vi "Integrl2.vi"(1 "Sampling frequency":i32=1000, 2 "Input Array":dbl[](array[numeric]) format="%.2f") -> (0 "Output Array (Integral)":dbl[](array[numeric]) format="%.2f")   [LabVIEW 2011]
uses:
  <vilib>/Analysis/NI_AALPro.lvlib
panel:
  out "Error":i32
  in  "Final condition":i32
  in  "Initial condition":i32
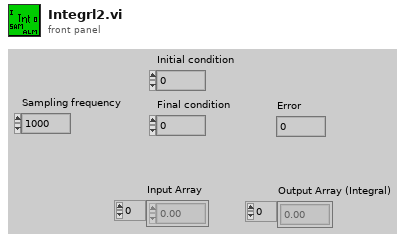
[diagram p1: front panel]
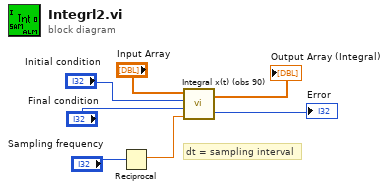
[diagram p0: block diagram]
diagram:
  # "dt = sampling interval"
  n1 = Reciprocal(x="Sampling frequency") -> (1/x=w3:dbl)
  n2 = call <vilib>:"Integral x(t) (obs 90).vi"("dt"=w3, "final condition"="Final condition", "initial condition"="Initial condition", "X"="Input Array") -> ("error"=→"Error":i32, "Integral X"=→"Output Array (Integral)":dbl[])
